vi "WPI_IMU_FGV.vi"(0 "SimpleGyroDevRef":T3 {"Sample Rate" min=0.25 max=100.0 step=0.25}, 1 "Operation":enum16{"set", "get"}(ring), 5 "Reset":bool, 7 "IMU Data":T2, 9 "IMU Angles":T1, 11 "IMU AHRS":cluster{"Pitch":dbl, "Roll":dbl, "Yaw":dbl}) -> (4 "SimpleGyroDevRef":T3 {"Sample Rate" min=0.25 max=100.0 step=0.25}, 6 "Reset Out":bool, 8 "IMU Data Out":T2, 10 "IMU Angles Out":T1, 15 "IMU AHRS Out":cluster{"Pitch":dbl, "Roll":dbl, "Yaw":dbl})   [LabVIEW 2015, in "FRC ADI MXP IMU.lvlib"]
uses:
  FRC ADI MXP IMU.lvlib
  WPI_AnalogDevicesIMUDevRef.ctl
  <vilib>/Rock Robotics/SystemInterfaces/spilib/spi_bus.ctl
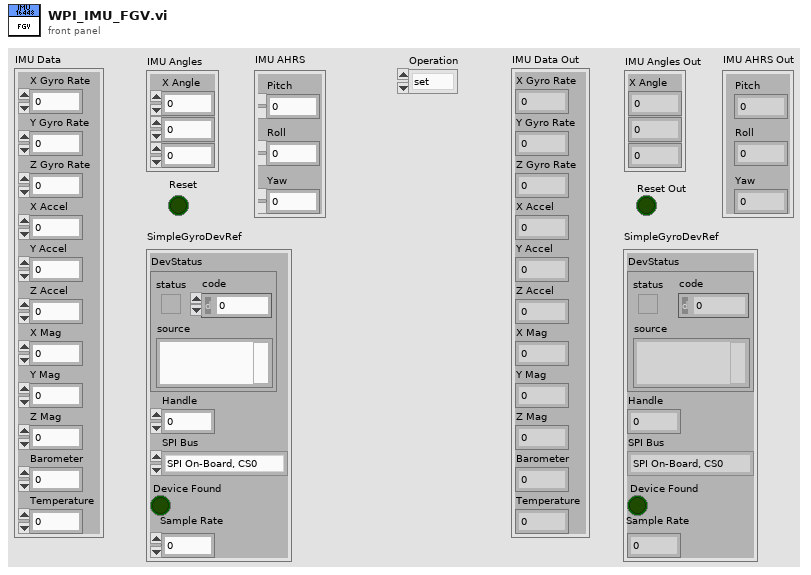
[diagram p1: front panel]
types:
  T1 = cluster{"X Angle":dbl, "Y Angle":dbl, "Z Angle":dbl}
  T2 = cluster{"X Gyro Rate":dbl, "Y Gyro Rate":dbl, "Z Gyro Rate":dbl, "X Accel":dbl, "Y Accel":dbl, "Z Accel":dbl, "X Mag":dbl, "Y Mag":dbl, "Z Mag":dbl, "Barometer":dbl, "Temperature":dbl}
  T3 = typedef "FRC ADI MXP IMU.lvlib/WPI_AnalogDevicesIMUDevRef.ctl" = cluster{"DevStatus":errorcluster, "Handle":i32, "SPI Bus":T4, "Device Found":bool, "Sample Rate":dbl}
  T4 = typedef "spi_bus.ctl" = enum16{"SPI On-Board, CS0", "SPI On-Board, CS1", "SPI On-Board, CS2", "SPI On-Board, CS3", "SPI MXP", "Invalid"}
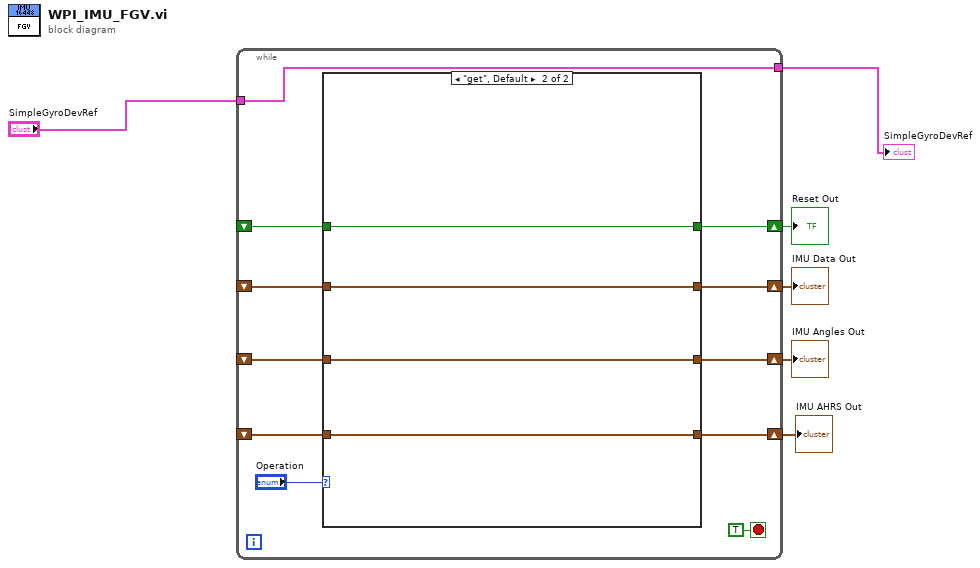
[diagram p0: block diagram]
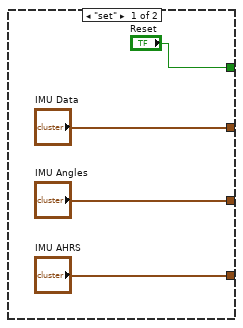
[diagram p2: hidden frame]
diagram:
  n1 = while {
    shift-right: [w15] -> w3
    shift-left: _ -> [w9]
    shift-right: [w14] -> w4
    shift-left: _ -> [w10]
    tunnel: "SimpleGyroDevRef" -> [w13]
    tunnel: [w13] -> w5
    shift-right: [w12] -> w2
    shift-left: _ -> [w11]
    shift-right: [w8] -> w1
    shift-left: _ -> [w7]
    stop <- TRUE stop-if-true
    n2 = case shown="\"get\", Default" "Operation" {
      tunnel: ["Reset" w23] -> w15
      tunnel: ["IMU Data" w24] -> w14
      tunnel: ["IMU Angles" w25] -> w12
      tunnel: w11 -> [_ w25]
      tunnel: w10 -> [_ w24]
      tunnel: w9 -> [_ w23]
      tunnel: ["IMU AHRS" w22] -> w8
      tunnel: w7 -> [_ w22]
      frame "set" {
      }
      frame "get", Default {
      }
    }
  }
  "SimpleGyroDevRef" <- w5
  "IMU Data Out" <- w4
  "Reset Out" <- w3
  "IMU Angles Out" <- w2
  "IMU AHRS Out" <- w1
